vi "Main.vi"(7 "GenNet Protocol":refnum<class "GenNet Protocol.lvclass">, 9 "Caller SystemMsg":refnum<user-event>, 10 "Caller MsgQ":refnum<class "DQMH-GenNet Message Queue.lvclass">, 11 "Module Admin":refnum<class "Delacor_lib_QMH_Cloneable Module Admin.lvclass">) -> ()   [LabVIEW 2020, in "GenNet-Client.lvlib"]
doc: "The GenNet-Client module is instantiated from a DQMH Generic Networking Module\nin order to forward messages via TCP/IP.\n\nThe GenNet-Client module forwards all requests to another DQMH Generic Networking \nModule running in another application and/or another PC accessible via TCP/IP.\n\n<b>Note:</b> This VI was modified by the <b>Validate DQMH Module</b> tool to upgrade it to the DQMH 5.0 approach to destroying cloneable module event references.\n\n<b>Note:</b> This VI was modified by the <b>Validate DQMH Module</b> tool to have the module name be passed as the Additional Information parameter with an Error Reported broadcast.\n\n<b>Note:</b> This VI was modified by the <b>Validate DQMH Module</b> tool to call the Release Message Queue VI in the top-level Error case.\n\n<b>Note:</b> This VI was modified by the <b>Validate DQMH Module</b> tool to call the Release Message Queue VI in the top-level Error case.\n\n<b>Note:</b> This VI was modified by the <b>Validate DQMH Module</b> tool to add a call to the Error Reported VI at the end of the 'Exit' MHL frame.\n\n____\nHAMPEL SOFTWARE ENGINEERING v3.8.0 (2023-12-18 14:41)"
uses:
  GenNet-Client.lvlib
  <vilib>/Delacor/Delacor QMH/Libraries/Cloneable Module Admin_class/Delacor_lib_QMH_Cloneable Module Admin.lvclass
  C:/Program Files (x86)/National Instruments/LabVIEW 2020/vi.lib/Delacor/Delacor QMH/Libraries/Module Admin_class/Delacor_lib_QMH_Module Admin.lvclass
  DQMH-GenNet Message Queue.lvclass
  hse-dqmh/Controls/System Message Argument--cluster.ctl
  hse-dqmh/Controls/System Message Source.ctl
  GenNet Protocols/GenNet Protocol.lvclass
  Module Data--cluster.ctl
  Stop Argument--cluster.ctl
  <vilib>/Delacor/Delacor QMH/Libraries/Message Queue_class/Delacor_lib_QMH_Message Queue.lvclass/Delacor_lib_QMH_Message Queue.ctl
  <vilib>/Delacor/Delacor QMH/Libraries/Cloneable Module Admin_class/Delacor_lib_QMH_Cloneable Module Admin.lvclass/Delacor_lib_QMH_Cloneable Module Admin.ctl
  <vilib>/Delacor/Delacor QMH/Libraries/Module Admin_class/Delacor_lib_QMH_Module Admin.lvclass/Delacor_lib_QMH_Module Admin.ctl
  Connect Argument--cluster.ctl
  Connect (Reply Payload)--cluster.ctl
  Send via Network Argument--cluster.ctl
  Listen for Network Broadcasts Argument--cluster.ctl
  <vilib>/Utility/miscctls.llb/LVPointTypeDef.ctl
  <vilib>/Delacor/Delacor QMH/Libraries/Message Queue_class/Delacor_lib_QMH_Enqueue Message (Single).vi
  <vilib>/Delacor/Delacor QMH/Libraries/Cloneable Module Admin_class/Delacor_lib_QMH_Get Module ID.vi
  <vilib>/Delacor/Delacor QMH/Libraries/Module Admin_class/Delacor_lib_QMH_Get External Launch.vi
  <vilib>/Utility/tcp.llb/UDP Multicast Read-Only Open.vi
  <vilib>/Utility/error.llb/Error Cluster From Error Code.vi
  <vilib>/ErrorRing/Error Ring.xnode
  <vilib>/Delacor/Delacor QMH/Libraries/Message Queue_class/Delacor_lib_QMH_Message Queue.lvclass
  hse-dqmh/hse-dqmh.lvlib
  hse-gennet.lvlib
panel:
  out "error out":errorcluster
  # "The GenNet Protocol allows for injecting the actual protocol (or, rather, the format\nor encoding used for the TCP messages). This also defines how to handle incoming\nmessages (eg. write them directly to the Caller MsgQ or broadcast them)"
  # "The GenNet-Client module is instantiated from a DQMH Generic Networking Module\nin order to forward messages via TCP/IP.\n\nThe GenNet-Client module forwards all requests to another DQMH Generic Networking \nModule running in another application and/or another PC accessible via TCP/IP."
  # "Caveat:\nThe Caller's message queue, which should be private to the caller only, is avail-\nable to the GenNet-Server module so that it can write messages directly. As the GenNet-Server\nmodule cannot be accessed from other code, and as messages that arrive via\nnetwork are to be considered local, this excemption to the rule is tolerable."
  # "Please get in touch with us at office@hampel-soft.com or visit our website www.hampel-soft.com"
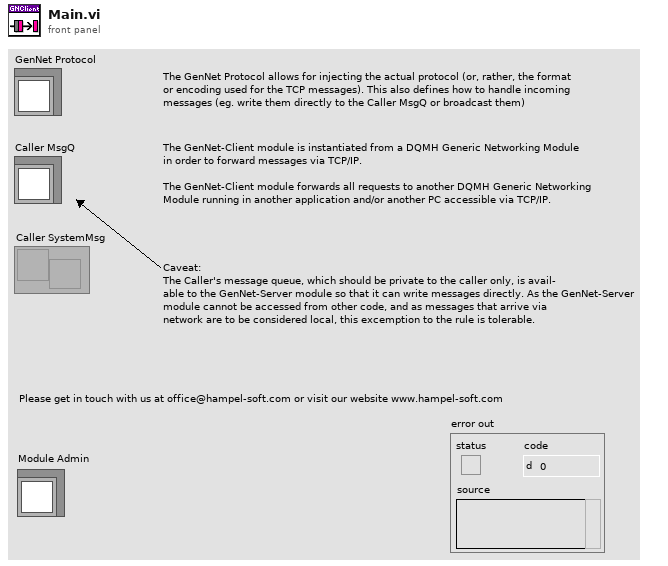
[diagram p1: front panel]
types:
  T1 = typedef "GenNet-Client.lvlib/Request Events--cluster.ctl" = cluster{"Stop Module":refnum<user-event>, "Show Panel":refnum<user-event>, "Hide Panel":refnum<user-event>, "Show Diagram":refnum<user-event>, "Get Module Execution Status":refnum<user-event>, "Send via Network":refnum<user-event>, "Connect":refnum<user-event>, "Listen for Network Broadcasts":refnum<user-event>}
  T2 = typedef "GenNet-Client.lvlib/Module Data--cluster.ctl" = cluster{"Status":string, "IP":string, "Port":u16, "Timeout":i32, "UDP ConnID":refnum<k16>, "TCP error":errorcluster, "GenNet Protocol":refnum<class "GenNet Protocol.lvclass">}
  T3 = enum32{"invalid lock state", "Not Locked", "Locked (No Password)", "Password-protected"}
  T4 = typedef "GenNet-Client.lvlib/Stop Argument--cluster.ctl" = cluster{"Origin":string, "Module ID":i32, "Exit via Stop Module Req?":bool, "Wait for Module to stop?":bool}
  T5 = typedef "GenNet-Client.lvlib/Connect Argument--cluster.ctl" = cluster{"Module ID":i32, "Wait Notifier":refnum<notifier>}
  T6 = typedef "GenNet-Client.lvlib/Send via Network Argument--cluster.ctl" = cluster{"Module ID":i32, "Message Data":variant}
  T7 = typedef "hse-dqmh.lvlib/System Message Argument--cluster.ctl" = cluster{"Identifier":string, "Payload":variant, "Sys. Msg. Source":T8, "Sys. Msg. Origin":string}
  T8 = typedef "hse-dqmh.lvlib/System Message Source.ctl" = enum16{"module", "application", "network"}
  T9 = typedef "GenNet-Client.lvlib/Listen for Network Broadcasts Argument--cluster.ctl" = cluster{"Module ID":i32, "Multicast Address":string, "Port":u16, "Local IP Address":string, "Max Rx Byte Size":i32}
  T10 = typedef "LVPointTypeDef.ctl" = cluster{"Horizontal":i16, "Vertical":i16}
  T11 = enum32{"Invalid", "Standard", "Closed", "Hidden", "Minimized", "Maximized"}
  T12 = typedef "GenNet-Client.lvlib/Connect (Reply Payload)--cluster.ctl" = cluster{"error":errorcluster, "Module ID":i32}
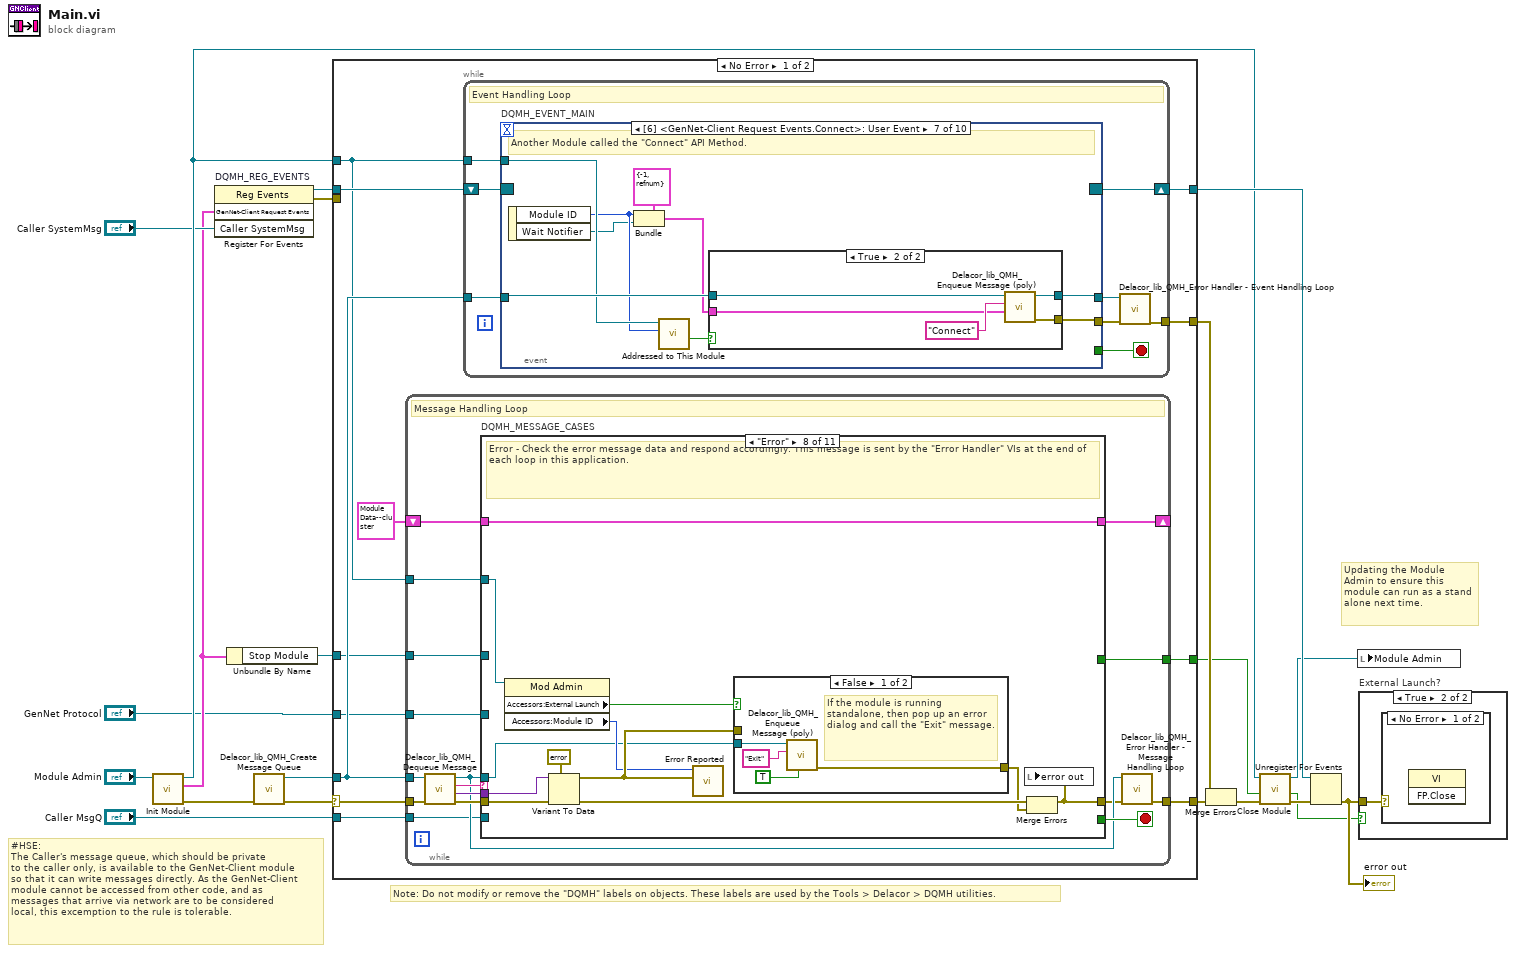
[diagram p0: block diagram]
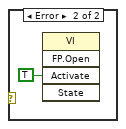
[diagram p3: hidden frame]
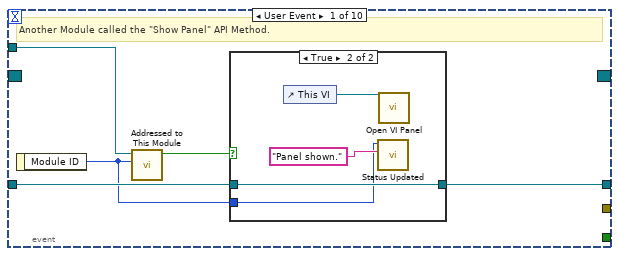
[diagram p4: hidden frame]
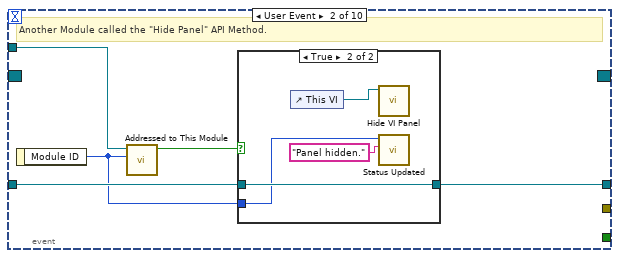
[diagram p6: hidden frame]
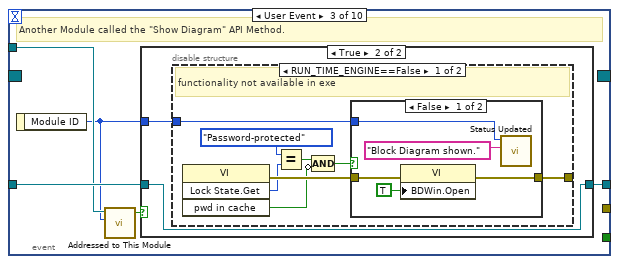
[diagram p8: hidden frame]
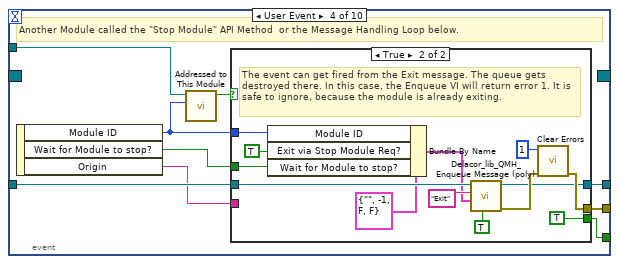
[diagram p12: hidden frame]
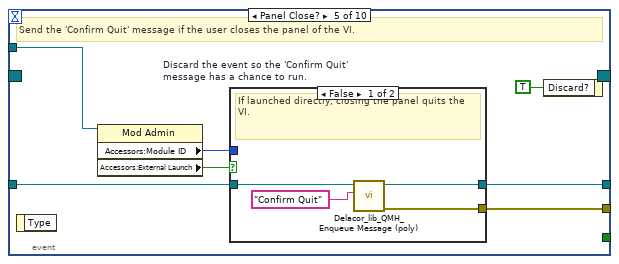
[diagram p14: hidden frame]
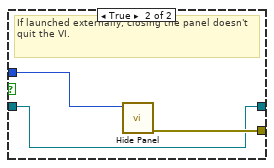
[diagram p15: hidden frame]
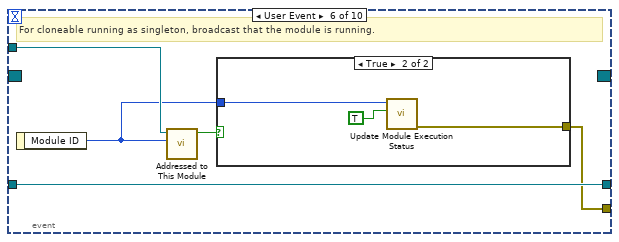
[diagram p16: hidden frame]
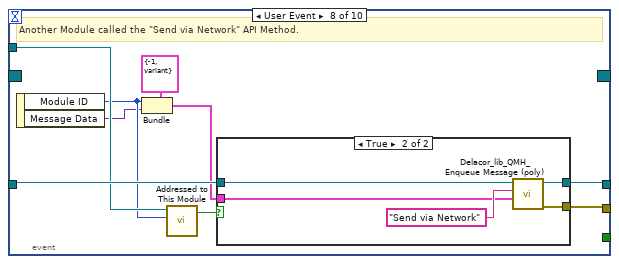
[diagram p19: hidden frame]
diagram:
  # "#HSE: \nThe Caller's message queue, which should be private \nto the caller only, is available to the GenNet-Client module \nso that it can write messages directly. As the GenNet-Client\nmodule cannot be accessed from other code, and as \nmessages that arrive via network are to be considered \nlocal, this excemption to the rule is tolerable."
  # "Note: Do not modify or remove the \"DQMH\" labels on objects. These labels are used by the Tools > Delacor > DQMH utilities."
  # "Updating the Module Admin to ensure this module can run as a stand alone next time."
  n1 = call "Init Module.vi"("Cloneable Module Admin in"="Module Admin") -> ("error out"=w18:errorcluster, "GenNet-Client Request Events"=w3:T1, "Cloneable Module Admin out"=w12:refnum<class "Delacor_lib_QMH_Cloneable Module Admin.lvclass">)  [unwired: 8 in]
  n2 = register-events "DQMH_REG_EVENTS"(w3, "Caller SystemMsg") -> (reference out=w16:refnum<event-registration>, error out=w5:errorcluster)  [unwired: 2 in]
  n3 = Unbundle By Name(w3) -> ("Stop Module"=w2:refnum<user-event>)
  n4 = call <vilib>:"Delacor_lib_QMH_Create Message Queue.vi"("error in"=w18) -> ("error out"=w7:errorcluster, "Message Queue"=w15:refnum<class "Delacor_lib_QMH_Message Queue.lvclass">)  [unwired: 9 in]
  n5 = case shown="No Error" w7 {
    selector: w7 -> [w27 w372]
    tunnel: [w33 w372] -> w19
    tunnel: [w32 w373] -> w17
    tunnel: w16 -> [w30 w373]
    tunnel: w15 -> [w29 w365]
    tunnel: [w28 _] -> w20
    tunnel: w12 -> [w26 w368]
    tunnel: [w25 _] -> w10
    tunnel: "Caller MsgQ" -> [w24 w364]
    tunnel: w5 -> [_ _]
    tunnel: w2 -> [w23 _]
    tunnel: "GenNet Protocol" -> [w22 _]
    frame No Error {
      n6 = while {
        tunnel: w29 -> [w210]
        shift-right: [w216] -> _
        shift-left: T2 {"Status"="", "IP"="", "Port"=0, "Timeout"=0, "UDP ConnID"=refnum, "TCP error"={"status"=FALSE, "code"=0, "source"=""}, "GenNet Protocol"=refnum} ("Data Cluster") -> [w203]
        tunnel: w27 -> [w214]
        tunnel: [w208] -> w33
        tunnel: w26 -> [w207]
        tunnel: [w206] -> w25
        tunnel: w24 -> [w205]
        tunnel: w23 -> [w202]
        tunnel: w22 -> [w201]
        stop <- w215 stop-if-true
        # "Message Handling Loop"
        n7 = call-dynamic "Delacor_lib_QMH_Dequeue Message.vi"("error in"=w214, "Message Queue in"=w210) -> ("error out"=w213:errorcluster, "Message Data"=w211:variant, "Message"=w212:string, "Message Queue out"=w209:refnum<class "Delacor_lib_QMH_Message Queue.lvclass">)  [unwired: 6 in]
        n8 = case "DQMH_MESSAGE_CASES" shown="\"Error\"" w212 {
          selector: w212 -> [_ _ _ _ _ _ _ _ _ _ w353]
          tunnel: w209 -> [_ _ _ _ _ _ _ w304 w322 w347 _]
          tunnel: w213 -> [w225 w240 w248 w275 w296 w299 w302 w313 w321 w349 _]
          tunnel: [w217 w238 w250 w268 w278 w297 w300 w303 w320 w333 w354] -> w204
          tunnel: w203 -> [w218 w239 w245 w267 w291 w298 w301 w312 w325 w334 w355]
          tunnel: [w218 w239 w246 w272 w290 w298 w301 w312 w325 w336 w355] -> w216
          tunnel: [_ _ _ _ _ _ _ _ _ w346 _] -> w215
          tunnel: w211 -> [_ _ w254 w274 w295 _ _ w311 _ w341 _]
          tunnel: w207 -> [w221 _ w257 _ w284 _ _ w308 _ w332 w351]
          tunnel: [_ _ _ _ _ _ _ _ _ w339 _] -> w206
          tunnel: w205 -> [_ _ w243 w269 w285 _ _ _ _ _ _]
          tunnel: w202 -> [_ _ _ _ w286 _ _ _ _ _ _]
          tunnel: w201 -> [_ _ w241 _ _ _ _ _ _ _ _]
          frame "Initialize" {
            # "Initialize - Any operation that needs to be done before the module can receive messages. Synchronize Caller Events.vi will inform Start Module.vi that the module has launched and is ready to receive messages. Module Did Init.vi will broadcast that the module initialized."
            n9 = call "Synchronize Caller Events.vi"("error in (no error)"=w225, "Module Admin"=w221) -> ("error out"=w223:errorcluster, "Module Admin out"=w220:refnum<class "Delacor_lib_QMH_Cloneable Module Admin.lvclass">)  [unwired: 8 in]
            n10 = property class="Mod Admin"(reference=w220) -> ("Accessors:Module ID"=w219:i32, "Accessors:External Launch"=w222:bool)  [unwired: 1 in, 2 out]
            n11 = call "Module Name--constant.vi"("Module ID"=w219) -> ("Module Name"=w226:string)  [unwired: 10 in]
            n12 = call "Module Did Init.vi"("error in (no error)"=w223, "Initialized?"=TRUE, "Origin"=w226, "Module ID"=w219) -> ("error out"=w217:errorcluster)  [unwired: 7 in]
            n13 = disable-structure shown="TARGET_TYPE==Windows||EMBEDDED_UI==True" {
              disable-tunnel: w219 -> [w229 _]
              disable-tunnel: w222 -> [w227 _]
              frame condition #0 (active) {
                n14 = call "Module Name--constant.vi"("Module ID"=w229) -> ("Module Name"=w233:string)  [unwired: 10 in]
                n15 = property class="VI"("Front Panel.Title"=w233) -> (reference out=w236:refnum<vi>, error out=w237:errorcluster)  [unwired: 2 in]
                n16 = Select(t=T11."Hidden" ("State"), s=w227, f=T11."Standard" ("State")) -> (s? t:f=w230:T11)
                n17 = invoke class="VI" method="FP.Open"(reference=w236, error in=w237, "State"=w230) -> (reference out=w235:refnum<vi>, error out=w234:errorcluster)  [unwired: 2 in, 3 out]
                n18 = invoke class="VI" method="FP.Center"(reference=w235, error in=w234) -> ()  [unwired: 1 in, 3 out]
                n19 = property on="Pane" class="Pane"("Origin"=T10 {"Horizontal"=0, "Vertical"=0}) -> ()  [unwired: 2 in, 2 out]
              }
              frame condition #1 {
              }
            }
          }
          frame "--- Module Specific ---" {
            # "Separator -- The following cases handle messages specific to this Module."
            n20 = Merge Errors(w240) -> (w238:errorcluster)
          }
          frame "Connect" {
            # "Open the TCP/IP connection to the GenNet Server"
            n21 = Variant To Data(error in=w248, type=T5 {"Module ID"=-1, "Wait Notifier"=refnum} ("Connect Argument"), Variant=w254) -> (data=w255:T5, error out=w247:errorcluster)
            n22 = property class="Mod Admin"(reference=w257) -> ("Accessors:Module ID"=w244:i32)  [unwired: 1 in, 2 out]
            n23 = Unbundle By Name(w255) -> ("Wait Notifier"=w258:refnum<notifier>)
            n24 = call "Establish Connection.vi"("GenNet Protocol"=w241, "error in"=errorcluster {"status"=FALSE, "code"=0, "source"=""}, "Caller's Queue In"=w243, "Module ID"=w244, "Data Cluster"=w245) -> ("error out"=w251:errorcluster, "Data Cluster out"=w246:T2)  [unwired: 5 in]
            n25 = Bundle By Name(cluster=T12 {"error"={"status"=FALSE, "code"=0, "source"=""}, "Module ID"=0} ("Connect (Reply Payload)"), "error"=w251, "Module ID"=w244) -> (w253:T12)
            n26 = Send Notification(notification=w253, notifier=w258) -> (error out=w249:errorcluster)  [unwired: 1 in, 1 out]
            n27 = Merge Errors(w247, w249) -> (w250:errorcluster)
          }
          frame "Send via Network" {
            # "Forwards the message of a DQMH module via Network"
            n28 = Variant To Data(error in=w275, type=T6 {"Module ID"=-1, "Message Data"=variant} ("Send via Network Argument"), Variant=w274) -> (data=w263:T6, error out=w270:errorcluster)
            n29 = Unbundle By Name(w267) -> ("IP"=w264:string, "Port"=w265:u16, "Timeout"=w266:i32)
            n30 = Unbundle By Name(w263) -> ("Message Data"=w260:variant)
            n31 = call "GetNet-Client Check Network Parameters.vi"("error in (no error)"=w270, "Timeout"=w266, "Port"=w265, "IP"=w264) -> ("error out"=w271:errorcluster)  [unwired: 7 in]
            n32 = call "GetNet-Client Send Message.vi"("error in"=w271, "Message Data"=w260, "Data Cluster in"=w267) -> ("error out"=w262:errorcluster, "Return Message Data"=w259:variant, "Data Cluster out"=w272:T2)  [unwired: 6 in]
            n33 = call "GenNet-Client Send Notification.vi"("error in"=w262, "Original Message Data"=w260, "Received Message Data"=w259) -> ("error out"=w261:errorcluster)  [unwired: 8 in]
            n34 = call "GenNet-Client Report Error.vi"("Caller MsgQ"=w269, "error in"=w261) -> ("error out"=w268:errorcluster)  [unwired: 9 in]
          }
          frame "Listen for Network Broadcasts" {
            # "Opens a port to listen for broadcasts sent by other modules via UDP"
            n35 = Variant To Data(error in=w296, type=T9 {"Module ID"=-1, "Multicast Address"="", "Port"=0, "Local IP Address"="", "Max Rx Byte Size"=10000} ("Listen for Network Broadcasts Argument"), Variant=w295) -> (data=w293:T9, error out=w279:errorcluster)
            n36 = property class="Mod Admin"(reference=w284) -> ("Accessors:Module ID"=w283:i32)  [unwired: 1 in, 2 out]
            n37 = Unbundle By Name(w293) -> ("Max Rx Byte Size"=w276:i32, "Local IP Address"=w277:string, "Port"=w280:u16, "Multicast Address"=w281:string)
            n38 = String To IP(1:w277) -> (0:w292:u32)
            n39 = String To IP(1:w281) -> (0:w289:u32)
            n40 = call-poly <vilib>:"UDP Multicast Open.vi"("net address"=w292, "error in (no error)"=w279, "multicast addr"=w289, "port"=w280) -> ("error out"=w287:errorcluster, "connection ID"=w288:refnum<k16>)  [unwired: 5 in, 1 out]
            n41 = call "NET-RX Spawn UDP Service.vi"("Max Rx Byte Size"=w276, "Module ID"=w283, "error in"=w287, "Caller MsgQ"=w285, "Stop Module"=w286, "UDP Connection ID"=w288) -> ("error out"=w278:errorcluster)  [unwired: 5 in]
            n42 = Bundle By Name(cluster=w291, "UDP ConnID"=w288) -> (w290:T2)
            n43 = Format Into String(format string="UDP Receiver created on Port %d and IP %s, Max Rx Byte Size = %d", w280, w281, w276) -> ()  [unwired: 2 in, 2 out]
          }
          frame "---Copy This Frame---" {
            # "Duplicate this frame when creating new messages.  Change this comment in the duplicated frame to describe this message."
            n44 = Merge Errors(w299) -> (w297:errorcluster)
          }
          frame "--- Exit and Error Handling---" {
            # "Separator - the following cases handle errors and exit messages."
            n45 = Merge Errors(w302) -> (w300:errorcluster)
          }
          frame "Error" {
            # "Error - Check the error message data and respond accordingly. This message is sent by the \"Error Handler\" VIs at the end of each loop in this application."
            n46 = property class="Mod Admin"(reference=w308) -> ("Accessors:External Launch"=w305:bool, "Accessors:Module ID"=w307:i32)  [unwired: 1 in, 2 out]
            n47 = Variant To Data(error in=w313, type=errorcluster {"status"=FALSE, "code"=0, "source"=""} ("error constant"), Variant=w311) -> (data=w314:errorcluster, error out=w309:errorcluster)
            n48 = call "Error Reported.vi"("Error"=w314, "Module ID"=w307) -> ()  [unwired: 9 in, 1 out]
            n49 = case shown="False" w305 {
              tunnel: [w318 _] -> w306
              tunnel: w304 -> [w317 _]
              tunnel: w314 -> [_ _]
              frame False {
                # "If the module is running standalone, then pop up an error dialog and call the \"Exit\" message."
                n50 = call-poly <vilib>:"Delacor_lib_QMH_Enqueue Message (poly).vi"("Priority Message? (F)"=TRUE, "Message"="Exit", "Message Queue in"=w317) -> ("error out"=w318:errorcluster)  [unwired: 7 in, 1 out]
              }
              frame True {
                # "If the module was launched externally, calling the Error Reported broadcast VI is the only action performed by the \"Error\" message. The module's caller can then process the error appropriately."
              }
            }
            n51 = Merge Errors(w309, w306) -> (w303:errorcluster)
            n52 = local write "error out"(w303) -> ()
          }
          frame "Confirm Quit" {
            # "#CodeNeeded - If you want to provide an \"Are you sure\" dialog (or some other notification) before the application exits, place that code here. This message is typically sent from a Panel Close? event."
            # "Confirm Quit - Message that can confirm whether or not the user wants to exit this instance."
            n53 = call-poly <vilib>:"Delacor_lib_QMH_Enqueue Message (poly).vi"("Priority Message? (F)"=TRUE, "error in"=w321, "Message"="Exit", "Message Queue in"=w322) -> ("error out"=w324:errorcluster)  [unwired: 6 in, 1 out]
            n54 = Merge Errors(w324) -> (w320:errorcluster)
          }
          frame "Exit" {
            w343 = 91  # 91: not all Exit messages will have an argument
            w346 = TRUE  # Stop the VI
            # "Release the message queue reference"
            # "Exit - Exit the application."
            n55 = Unbundle By Name(w334) -> ("GenNet Protocol"=w337:refnum<class "GenNet Protocol.lvclass">, "UDP ConnID"=w329:refnum<k16>)
            n56 = Variant To Data(error in=w349, type=T4 {"Origin"="", "Module ID"=-1, "Exit via Stop Module Req?"=FALSE, "Wait for Module to stop?"=FALSE} ("Stop Argument"), Variant=w341) -> (data=w331:T4, error out=w342:errorcluster)
            n57 = call-dynamic "Close Connection.vi"("GenNet Protocol in"=w337) -> ("GenNet Protocol out"=w335:refnum<class "GenNet Protocol.lvclass">)  [unwired: 9 in, 1 out]
            n58 = call "GenNet Close UDP Connection.vi"("UDP Network Connection in"=w329) -> ("UDP Network Connection out"=w330:refnum<k16>)  [unwired: 9 in, 1 out]
            n59 = call <vilib>:"Clear Errors.vi"("error in (no error)"=w342, "specific error code to clear (0: all)"=w343) -> ("error out"=w348:errorcluster)  [unwired: 4 in, 1 out]
            n60 = control-ref of="This VI"() -> (w338:refnum<vi>)
            n61 = Bundle By Name(cluster=w334, "GenNet Protocol"=w335, "UDP ConnID"=w330) -> (w336:T2)
            n62 = call "Handle Exit.vi"("Stop Argument"=w331, "Module Admin in"=w332, "VI reference"=w338) -> ("error out"=w344:errorcluster, "Wait for Stop?"=w339:bool)  [unwired: 7 in]
            n63 = call-dynamic "Delacor_lib_QMH_Release Message Queue.vi"("error in"=w348, "Message Queue"=w347) -> ("error out"=w345:errorcluster)  [unwired: 9 in]
            n64 = property class="Mod Admin"(reference=w332) -> ("Accessors:Module ID"=w326:i32)  [unwired: 1 in, 2 out]
            n65 = Merge Errors(w344, w345) -> (w333:errorcluster)
            n66 = Unbundle By Name(w331) -> ()  [unwired: 1 out]
            n67 = property class="Mod Admin"(reference=w332) -> ("Accessors:Module ID"=w327:i32)  [unwired: 1 in, 2 out]
            n68 = call "Error Reported.vi"("Error"=w333, "Module ID"=w326) -> ()  [unwired: 9 in, 1 out]
            n69 = call "Status Updated.vi"("Status"="Client disconnected and exited." ("Message"), "Module ID"=w327) -> ()  [unwired: 9 in, 1 out]
          }
          frame Default {
            # "'Default' case only runs if there is a message that isn't defined in any of the other cases.  Output a programming error."
            n70 = property class="Mod Admin"(reference=w351) -> ("Accessors:Module ID"=w350:i32)  [unwired: 1 in, 2 out]
            n71 = call "Module Name--constant.vi"("Module ID"=w350) -> ("Module Name"=w352:string)  [unwired: 10 in]
            n72 = xnode "Error Ring"("parameter 0"=w353, "parameter 1"=w352) -> ("error out"=w354:errorcluster)
          }
        }
        n73 = call-dynamic "Delacor_lib_QMH_Error Handler - Message Handling Loop.vi"("error in"=w204, "Message Queue in"=w209) -> ("dup error in"=w208:errorcluster)  [unwired: 8 in, 1 out]
      }
      n74 = while {
        tunnel: w29 -> [w41]
        shift-right: [w39] -> w32
        shift-left: w30 -> [w40]
        tunnel: [w35] -> w28
        tunnel: w26 -> [w34]
        stop <- w37 stop-if-true
        # "Event Handling Loop"
        n75 = event "DQMH_EVENT_MAIN" shown="[6] <GenNet-Client Request Events.Connect>: User Event" {
          selector: w40 -> [_ _ _ _ _ _ _ _ _ _]
          dyn-events: [_ _ _ _ _ _ _ _ _ _] -> w39
          timeout: _ -> [_ _ _ _ _ _ _ _ _ _]
          tunnel: [_ _ _ w87 _ _ _ _ _ _] -> w37
          tunnel: w41 -> [w46 w56 w66 w90 w112 w123 w137 w152 w165 w194]
          tunnel: [_ _ _ w92 w111 w122 w129 w144 w163 w185] -> w38
          tunnel: [w45 w55 w65 w91 w110 w123 w136 w151 w164 w193] -> w36
          tunnel: w34 -> [w43 w53 w63 w89 w109 w124 w134 w149 _ w191]
          event User Event {
            # "Another Module called the \"Show Panel\" API Method."
            n76 = event-data() -> ("Module ID"=w42:i32)  [unwired: 1 in]
            n77 = call "Addressed to This Module.vi"("Module ID from Argument"=w42, "Module Admin"=w43) -> ("Addressed to this instance?"=w44:bool)  [unwired: 8 in, 1 out]
            n78 = case shown="True" w44 {
              tunnel: w46 -> [w47 w51]
              tunnel: [w47 w51] -> w45
              tunnel: w42 -> [_ w48]
              frame False {
              }
              frame True {
                n79 = control-ref of="This VI"() -> (w49:refnum<vi>)
                n80 = call "Status Updated.vi"("Status"="Panel shown." ("format string"), "Module ID"=w48) -> ()  [unwired: 9 in, 1 out]
                n81 = call "Open VI Panel.vi"("VI"=w49) -> ()  [unwired: 10 in, 1 out]
              }
            }
          }
          event User Event {
            # "Another Module called the \"Hide Panel\" API Method."
            n82 = event-data() -> ("Module ID"=w52:i32)  [unwired: 1 in]
            n83 = call "Addressed to This Module.vi"("Module ID from Argument"=w52, "Module Admin"=w53) -> ("Addressed to this instance?"=w54:bool)  [unwired: 8 in, 1 out]
            n84 = case shown="True" w54 {
              tunnel: w56 -> [w57 w61]
              tunnel: [w57 w61] -> w55
              tunnel: w52 -> [_ w59]
              frame False {
              }
              frame True {
                n85 = control-ref of="This VI"() -> (w58:refnum<vi>)
                n86 = call "Hide VI Panel.vi"("VI"=w58) -> ()  [unwired: 10 in, 1 out]
                n87 = call "Status Updated.vi"("Status"="Panel hidden." ("format string"), "Module ID"=w59) -> ()  [unwired: 9 in, 1 out]
              }
            }
          }
          event User Event {
            # "Another Module called the \"Show Diagram\" API Method."
            n88 = event-data() -> ("Module ID"=w62:i32)  [unwired: 1 in]
            n89 = call "Addressed to This Module.vi"("Module ID from Argument"=w62, "Module Admin"=w63) -> ("Addressed to this instance?"=w64:bool)  [unwired: 8 in, 1 out]
            n90 = case shown="True" w64 {
              tunnel: w66 -> [w67 w68]
              tunnel: [w67 w68] -> w65
              tunnel: w62 -> [_ w69]
              frame False {
              }
              frame True {
                n91 = disable-structure shown="RUN_TIME_ENGINE==False" {
                  disable-tunnel: [w77 _] -> _
                  disable-tunnel: w69 -> [w70 _]
                  frame condition #0 (active) {
                    # "functionality not available in exe"
                    n92 = invoke class="VI" method="Lock State.Get"() -> (error out=w76:errorcluster, "Get Lock State"=w75:T3, "pwd in cache"=w72:bool)  [unwired: 4 in, 1 out]
                    n93 = Equal?(x=T3."Password-protected", y=w75) -> (x = y?=w73:bool)
                    n94 = Compound Arithmetic op=AND(w73, invert w72) -> (w71:bool)
                    n95 = case shown="False" w71 {
                      tunnel: [w81 w83] -> w77
                      tunnel: w76 -> [w80 w83]
                      tunnel: w70 -> [w78 _]
                      frame False {
                        n96 = property class="VI"(error in=w80, "BDWin.Open"=TRUE ("Block Diagram Window:Open")) -> (error out=w81:errorcluster)  [unwired: 1 in, 1 out]
                        n97 = call "Status Updated.vi"("Status"="Block Diagram shown." ("format string"), "Module ID"=w78) -> ()  [unwired: 9 in, 1 out]
                      }
                      frame True {
                        # "Password-protected VI, and the password is not in the cache. Do not show the diagram."
                      }
                    }
                  }
                  frame condition #1 {
                  }
                }
              }
            }
          }
          event User Event {
            # "Another Module called the \"Stop Module\" API Method  or the Message Handling Loop below."
            n98 = event-data() -> ("Module ID"=w85:i32, "Wait for Module to stop?"=w86:bool, "Origin"=w84:string)  [unwired: 1 in]
            n99 = call "Addressed to This Module.vi"("Module ID from Argument"=w85, "Module Admin"=w89) -> ("Addressed to this instance?"=w88:bool)  [unwired: 8 in, 1 out]
            n100 = case shown="True" w88 {
              tunnel: [_ w102] -> w92
              tunnel: [w93 w101] -> w91
              tunnel: w90 -> [w93 w100]
              tunnel: [_ TRUE] -> w87
              tunnel: w86 -> [_ w95]
              tunnel: w85 -> [_ w97]
              tunnel: w84 -> [_ _]
              frame False {
              }
              frame True {
                # "The event can get fired from the Exit message. The queue gets destroyed there. In this case, the Enqueue VI will return error 1. It is safe to ignore, because the module is already exiting."
                n101 = Bundle By Name(cluster=T4 {"Origin"="", "Module ID"=-1, "Exit via Stop Module Req?"=FALSE, "Wait for Module to stop?"=FALSE} ("Stop Argument"), "Module ID"=w97, "Exit via Stop Module Req?"=TRUE, "Wait for Module to stop?"=w95) -> (w94:T4)
                n102 = call-poly <vilib>:"Delacor_lib_QMH_Enqueue Message (poly).vi"("Priority Message? (F)"=TRUE, "Message Data"=w94, "Message"="Exit", "Message Queue in"=w100) -> ("error out"=w105:errorcluster, "Message Queue out"=w101:refnum<class "Delacor_lib_QMH_Message Queue.lvclass">)  [unwired: 6 in]
                n103 = call <vilib>:"Clear Errors.vi"("error in (no error)"=w105, "specific error code to clear (0: all)"=1) -> ("error out"=w102:errorcluster)  [unwired: 4 in, 1 out]
              }
            }
          }
          event Panel Close? {
            w113 = TRUE  # Discard the event so the 'Confirm Quit' message has a chance to run.
            # "Send the 'Confirm Quit' message if the user closes the panel of the VI."
            n104 = event-data() -> ()  [unwired: 1 in, 1 out]
            n105 = property class="Mod Admin"(reference=w109) -> ("Accessors:Module ID"=w107:i32, "Accessors:External Launch"=w108:bool)  [unwired: 1 in, 2 out]
            n106 = case shown="False" w108 {
              tunnel: w112 -> [w117 w118]
              tunnel: [w116 w120] -> w111
              tunnel: [w115 w118] -> w110
              tunnel: w107 -> [_ w119]
              frame False {
                # "If launched directly, closing the panel quits the VI."
                n107 = call-poly <vilib>:"Delacor_lib_QMH_Enqueue Message (poly).vi"("Message"="Confirm Quit", "Message Queue in"=w117) -> ("error out"=w116:errorcluster, "Message Queue out"=w115:refnum<class "Delacor_lib_QMH_Message Queue.lvclass">)  [unwired: 8 in]
              }
              frame True {
                # "If launched externally, closing the panel doesn't quit the VI."
                n108 = call "Hide Panel.vi"("Module ID"=w119) -> ("error out"=w120:errorcluster)  [unwired: 10 in]
              }
            }
            n109 = event-data("Discard?"=w113) -> ()  [unwired: 1 in, 1 out]
          }
          event User Event {
            # "For cloneable running as singleton, broadcast that the module is running."
            n110 = event-data() -> ("Module ID"=w121:i32)  [unwired: 1 in]
            n111 = call "Addressed to This Module.vi"("Module ID from Argument"=w121, "Module Admin"=w124) -> ("Addressed to this instance?"=w125:bool)  [unwired: 8 in, 1 out]
            n112 = case shown="True" w125 {
              tunnel: [_ w128] -> w122
              tunnel: w121 -> [_ w127]
              frame False {
              }
              frame True {
                n113 = call "Update Module Execution Status.vi"("Running?"=TRUE, "Module ID"=w127) -> ("error out"=w128:errorcluster)  [unwired: 9 in]
              }
            }
          }
          event User Event {
            # "Another Module called the \"Connect\" API Method."
            n114 = event-data() -> ("Module ID"=w131:i32, "Wait Notifier"=w130:refnum<notifier>)  [unwired: 1 in]
            n115 = Bundle(cluster=T5 {"Module ID"=-1, "Wait Notifier"=refnum} ("Connect Argument"), "Module ID"=w131, "Wait Notifier"=w130) -> (w132:T5)
            n116 = call "Addressed to This Module.vi"("Module ID from Argument"=w131, "Module Admin"=w134) -> ("Addressed to this instance?"=w135:bool)  [unwired: 8 in, 1 out]
            n117 = case shown="True" w135 {
              tunnel: w137 -> [w138 w143]
              tunnel: [w138 w142] -> w136
              tunnel: w132 -> [_ w140]
              tunnel: [_ w139] -> w129
              frame False {
              }
              frame True {
                n118 = call-poly <vilib>:"Delacor_lib_QMH_Enqueue Message (poly).vi"("Message Data"=w140, "Message"="Connect", "Message Queue in"=w143) -> ("error out"=w139:errorcluster, "Message Queue out"=w142:refnum<class "Delacor_lib_QMH_Message Queue.lvclass">)  [unwired: 7 in]
              }
            }
          }
          event User Event {
            # "Another Module called the \"Send via Network\" API Method."
            n119 = event-data() -> ("Module ID"=w146:i32, "Message Data"=w145:variant)  [unwired: 1 in]
            n120 = Bundle(cluster=T6 {"Module ID"=-1, "Message Data"=variant} ("Send via Network Argument"), "Module ID"=w146, "Message Data"=w145) -> (w147:T6)
            n121 = call "Addressed to This Module.vi"("Module ID from Argument"=w146, "Module Admin"=w149) -> ("Addressed to this instance?"=w150:bool)  [unwired: 8 in, 1 out]
            n122 = case shown="True" w150 {
              tunnel: w152 -> [w153 w158]
              tunnel: [w153 w157] -> w151
              tunnel: w147 -> [_ w155]
              tunnel: [_ w154] -> w144
              frame False {
              }
              frame True {
                n123 = call-poly <vilib>:"Delacor_lib_QMH_Enqueue Message (poly).vi"("Message Data"=w155, "Message"="Send via Network", "Message Queue in"=w158) -> ("error out"=w154:errorcluster, "Message Queue out"=w157:refnum<class "Delacor_lib_QMH_Message Queue.lvclass">)  [unwired: 7 in]
              }
            }
          }
          event User Event {
            # "Caller triggered a \"System Message\" Broadcast Event"
            n124 = event-data() -> ("Sys. Msg. Origin"=w159:string, "Identifier"=w162:string, "Payload"=w161:variant, "Sys. Msg. Source"=w160:T8)  [unwired: 1 in]
            n125 = case shown="Default" w160 {
              tunnel: w165 -> [w166 w182]
              tunnel: [w166 w181] -> w164
              tunnel: [_ w180] -> w163
              tunnel: w162 -> [_ w176]
              tunnel: w161 -> [_ w175]
              tunnel: w159 -> [_ w167]
              frame "network" {
                # "do not forward messages from source \"network\""
              }
              frame Default {
                # "default: forward, and overwrite source with \"network\""
                n126 = Bundle(cluster=T7 {"Identifier"="", "Payload"=variant, "Sys. Msg. Source"=enum."module", "Sys. Msg. Origin"=""} ("System Message Argument"), "Identifier"=w176, "Payload"=w175, "Sys. Msg. Source"=System_Message_Source."network" ("Source"), "Sys. Msg. Origin"=w167) -> (w174:T7)
                n127 = To Variant(anything=w174) -> (Variant=w173:variant)
                n128 = Set Variant Attribute(Variant=w173, name="message", value="System Message" ("name")) -> (Variant out=w172:variant)  [unwired: 1 in, 2 out]
                n129 = Bundle By Name(cluster=T6 {"Module ID"=-1, "Message Data"=variant} ("Send via Network Argument"), "Message Data"=w172) -> (w177:T6)
                n130 = call-poly <vilib>:"Delacor_lib_QMH_Enqueue Message (poly).vi"("Message Data"=w177, "Message"="Send via Network", "Message Queue in"=w182) -> ("error out"=w180:errorcluster, "Message Queue out"=w181:refnum<class "Delacor_lib_QMH_Message Queue.lvclass">)  [unwired: 7 in]
              }
            }
          }
          event User Event {
            # "Another Module called the \"Listen for Network Broadcasts\" API Method."
            n131 = event-data() -> ("Module ID"=w188:i32, "Multicast Address"=w187:string, "Port"=w186:u16, "Local IP Address"=w184:string, "Max Rx Byte Size"=w183:i32)  [unwired: 1 in]
            n132 = Bundle(cluster=T9 {"Module ID"=-1, "Multicast Address"="", "Port"=0, "Local IP Address"="", "Max Rx Byte Size"=10000} ("Listen for Network Broadcasts Argument"), "Module ID"=w188, "Multicast Address"=w187, "Port"=w186, "Local IP Address"=w184, "Max Rx Byte Size"=w183) -> (w189:T9)
            n133 = call "Addressed to This Module.vi"("Module ID from Argument"=w188, "Module Admin"=w191) -> ("Addressed to this instance?"=w192:bool)  [unwired: 8 in, 1 out]
            n134 = case shown="True" w192 {
              tunnel: w194 -> [w195 w200]
              tunnel: [w195 w199] -> w193
              tunnel: w189 -> [_ w197]
              tunnel: [_ w196] -> w185
              frame False {
              }
              frame True {
                n135 = call-poly <vilib>:"Delacor_lib_QMH_Enqueue Message (poly).vi"("Message Data"=w197, "Message"="Listen for Network Broadcasts", "Message Queue in"=w200) -> ("error out"=w196:errorcluster, "Message Queue out"=w199:refnum<class "Delacor_lib_QMH_Message Queue.lvclass">)  [unwired: 7 in]
              }
            }
          }
        }
        n136 = call-dynamic "Delacor_lib_QMH_Error Handler - Event Handling Loop.vi"("error in"=w38, "Message Queue in"=w36) -> ("dup error in"=w35:errorcluster)  [unwired: 8 in, 1 out]
      }
    }
    frame Error {
      n137 = call "Synchronize Caller Events.vi"("Module Admin"=w368) -> ("Module Admin out"=w367:refnum<class "Delacor_lib_QMH_Cloneable Module Admin.lvclass">)  [unwired: 9 in, 1 out]
      n138 = property class="Mod Admin"(reference=w367) -> ("Accessors:Module ID"=w366:i32)  [unwired: 1 in, 2 out]
      n139 = call-dynamic "Delacor_lib_QMH_Release Message Queue.vi"("Message Queue"=w365) -> ()  [unwired: 10 in, 1 out]
      n140 = call-dynamic "Delacor_lib_QMH_Release Message Queue.vi"("Message Queue"=w364) -> ()  [unwired: 10 in, 1 out]
      n141 = call "Module Name--constant.vi"("Module ID"=w366) -> ("Module Name"=w371:string)  [unwired: 10 in]
      n142 = Format Into String(format string="An error occurred during initialization. %s is no longer running.", w371) -> (resulting string=w369:string)  [unwired: 2 in, 1 out]
      n143 = call "Error Reported.vi"("Additional Information"=w369, "Error"=w372, "Module ID"=w366) -> ()  [unwired: 8 in, 1 out]
    }
  }
  n144 = Merge Errors(w20, w19) -> (w21:errorcluster)
  n145 = call "Close Module.vi"("error in (no error)"=w21, "Wait for stop?"=w10, "Module Admin in"=w12) -> ("error out"=w14:errorcluster, "External Launch"=w8:bool, "Module Admin out"=w11:refnum<class "Delacor_lib_QMH_Cloneable Module Admin.lvclass">)  [unwired: 6 in]
  n146 = Unregister For Events(event registration refnum=w17, error in=w14) -> (error out=w9:errorcluster)
  "error out" <- w9
  n147 = local write "Module Admin"(w11) -> ()
  n148 = case "External Launch?" shown="True" w8 {
    tunnel: w9 -> [_ w374]
    frame False {
    }
    frame True {
      n149 = case shown="No Error" w374 {
        frame No Error {
          n150 = invoke class="VI" method="FP.Close"() -> ()  [unwired: 3 in, 3 out]
        }
        frame Error {
          n151 = invoke class="VI" method="FP.Open"("Activate"=TRUE ("Activate?")) -> ()  [unwired: 4 in, 5 out]
        }
      }
    }
  }
